vi "Untitled 4 (SubVI).vi"(8 "error in (no error)":errorcluster, 9 "data":variant, 10 "message":string, 11 "queueName":string) -> (0 "error out":errorcluster)   [LabVIEW 2018]
uses:
  Queue/QueueMessage.ctl
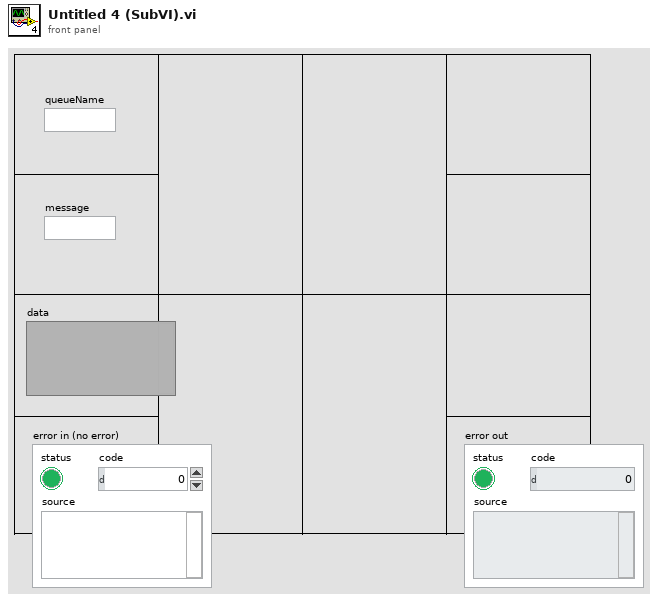
[diagram p1: front panel]
types:
  T1 = typedef "QueueMessage.ctl" = cluster{"message":string, "data":variant}
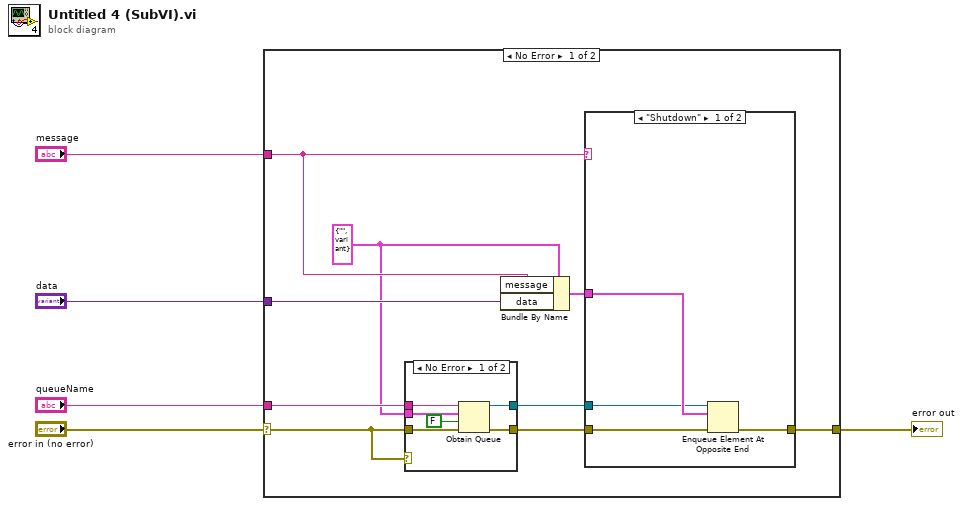
[diagram p0: block diagram]
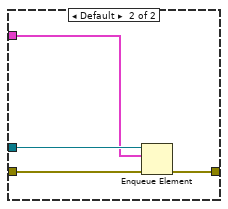
[diagram p3: hidden frame]
diagram:
  n1 = case shown="No Error" "error in (no error)" {
    selector: "error in (no error)" -> [w6 w29]
    tunnel: [w14 w29] -> w1
    tunnel: "queueName" -> [w12 _]
    tunnel: "message" -> [w10 _]
    tunnel: "data" -> [w11 _]
    frame No Error {
      w7 = T1 {"message"="", "data"=variant} ("QueueMessage")
      n2 = case shown="No Error" w6 {
        tunnel: w6 -> [w20 _]
        tunnel: [w19 _] -> w13
        tunnel: w12 -> [w18 _]
        tunnel: [w17 _] -> w8
        tunnel: w7 -> [w15 _]
        frame No Error {
          n3 = Obtain Queue(name (unnamed)=w18, element data type=w15, create if not found? (T)=FALSE, error in (no error)=w20) -> (queue out=w17:refnum<queue>, error out=w19:errorcluster)  [unwired: 1 in, 1 out]
        }
        frame Error {
        }
      }
      n4 = Bundle By Name(cluster=w7, "message"=w10, "data"=w11) -> (w9:T1)
      n5 = case shown="\"Shutdown\"" w10 {
        tunnel: w13 -> [w24 w28]
        tunnel: [w23 w27] -> w14
        tunnel: w9 -> [w22 w25]
        tunnel: w8 -> [w21 w26]
        frame "Shutdown" {
          n6 = Enqueue Element At Opposite End(queue=w21, element=w22, error in (no error)=w24) -> (error out=w23:errorcluster)  [unwired: 1 in, 2 out]
        }
        frame Default {
          n7 = Enqueue Element(queue=w26, element=w25, error in (no error)=w28) -> (error out=w27:errorcluster)  [unwired: 1 in, 2 out]
        }
      }
    }
    frame Error {
    }
  }
  "error out" <- w1
